vi "Active Chal.vi"(8 "error in (no error)":errorcluster, 11 "SOL-Config in":refnum<class "SOL-Config.lvclass">) -> (0 "error out":errorcluster, 2 "Active Chal":i64, 3 "SOL-Config out":refnum<class "SOL-Config.lvclass">)   [LabVIEW 2020, in "Summer of LabVIEW.lvlib" / "SOL-Config.lvclass"]
uses:
  SOL-Config.lvclass
  SOL-Config.lvclass/SOL-Config.ctl
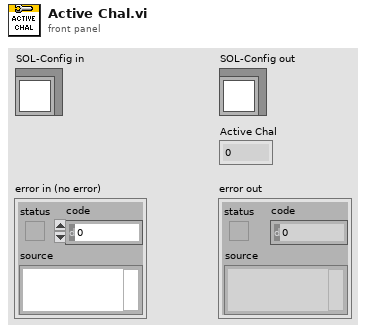
[diagram p1: front panel]
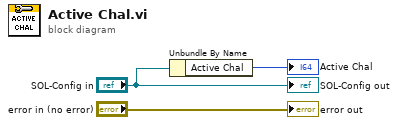
[diagram p0: block diagram]
diagram:
  n1 = Unbundle By Name("SOL-Config in") -> ("Active Chal"=→"Active Chal":i64)
  "error out" <- "error in (no error)"
  "SOL-Config out" <- "SOL-Config in"
